vi "HW_QX_FetchData.vi"(8 "Error in":errorcluster caption="error in", 10 "QX Cfg":T2[](array[typedef]), 11 "QXDAQ reference":refnum<k24>) -> (0 "error out":errorcluster, 2 "Data Out":T1[](array[typedef]))   [LabVIEW 2016]
uses:
  DAQ_ReadBlock.ctl
  QX Device Configuration.ctl
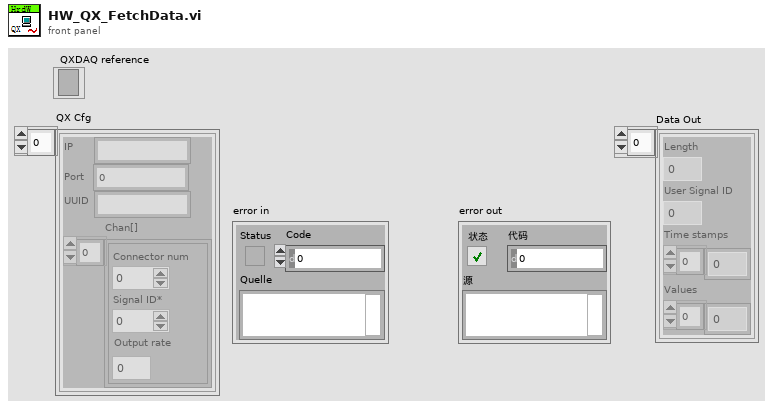
[diagram p1: front panel]
types:
  T1 = typedef "DAQ_ReadBlock.ctl" = cluster{"Length":i32, "User Signal ID":i32, "Time stamps":dbl[], "Values":dbl[]}
  T2 = typedef "QX Device Configuration.ctl" = cluster{"IP":string, "Port":i32, "UUID":string, "Chan[]":cluster{"Connector num":i32, "Signal ID*":i32, "Output rate":dbl}[]}
  T3 = cluster{"Connector num":i32, "Signal ID*":i32, "Output rate":dbl}[]
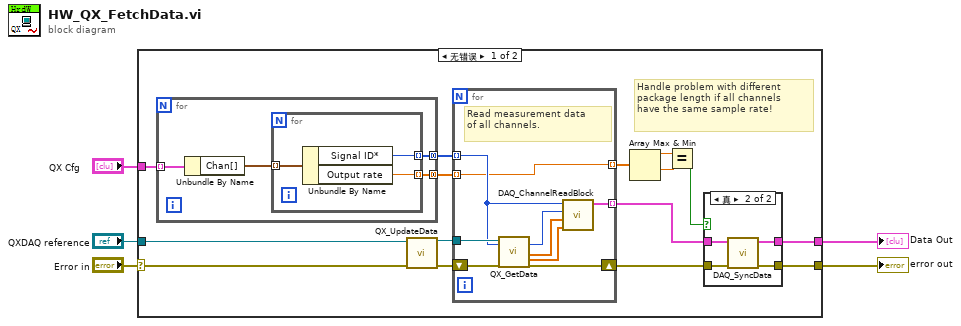
[diagram p0: block diagram]
diagram:
  n1 = case shown="无错误" "Error in" {
    selector: "Error in" -> [w10 w43]
    tunnel: "QX Cfg" -> [w13 _]
    tunnel: [w9 w43] -> w3
    tunnel: "QXDAQ reference" -> [w7 _]
    tunnel: [w6 _] -> w1
    frame No Error {
      # "Handle problem with different\npackage length if all channels\nhave the same sample rate!"
      n2 = for {
        tunnel: w13 -> [w24] mode=indexing
        tunnel: [w22] -> w12 mode=concatenating
        tunnel: [w21] -> w11 mode=concatenating
        n3 = Unbundle By Name(w24) -> ("Chan[]"=w23:T3)
        n4 = for {
          tunnel: w23 -> [w27] mode=indexing
          tunnel: [w26] -> w22 mode=indexing
          tunnel: [w25] -> w21 mode=indexing
          n5 = Unbundle By Name(w27) -> ("Signal ID*"=w26:i32, "Output rate"=w25:dbl)
        }
      }
      n6 = call <userlib>:"QX_UpdateData.vi"("Error in"=w10, "QXDAQ reference"=w7) -> ("Error out"=w20:errorcluster, "QXDAQ reference"=w19:refnum<k24>)  [unwired: 8 in]
      n7 = for {
        tunnel: w19 -> [w41]
        shift-right: [w40] -> w17
        shift-left: w20 -> [w42]
        tunnel: [w37] -> w18 mode=indexing
        tunnel: [w34] -> w8 mode=indexing
        tunnel: w12 -> [w35] mode=indexing
        tunnel: w11 -> [w34] mode=indexing
        # "Read measurement data\nof all channels."
        n8 = call <userlib>:"QX_GetData.vi"("QXDAQ reference"=w41, "UserSignalID"=w35, "Error in"=w42) -> ("Count"=w39:i32, "Time stamps"=w38:dbl[], "Values"=w36:dbl[], "Error out"=w40:errorcluster)  [unwired: 11 in, 2 out]
        n9 = call "DAQ_ChannelReadBlock.vi"("User Signal ID"=w35, "Count"=w39, "Time stamps"=w38, "Values"=w36) -> ("Read block"=w37:T1)  [unwired: 6 in]
      }
      n10 = Array Max & Min(array=w8) -> (max value=w15:dbl, min value=w16:dbl)  [unwired: 2 out]
      n11 = Equal?(x=w15, y=w16) -> (x = y?=w14:bool)
      n12 = case shown="真" w14 {
        tunnel: w18 -> [w29 w33]
        tunnel: w17 -> [w28 w32]
        tunnel: [w28 w31] -> w9
        tunnel: [w29 w30] -> w6
        frame False {
        }
        frame True {
          n13 = call "DAQ_SyncData.vi"("Fehler (Eingang)"=w32, "Data In"=w33) -> ("Fehler (Ausgang)"=w31:errorcluster, "Data Out"=w30:T1[])  [unwired: 6 in, 2 out]
        }
      }
    }
    frame Error {
    }
  }
  "error out" <- w3
  "Data Out" <- w1
